vi "Write Wavelength.vi"(8 "error in":errorcluster, 10 "Wavelength (nm)":dbl, 11 "LTB-1 in":refnum<class "LTB-1.lvclass">) -> (0 "error out":errorcluster, 3 "LTB-1 out":refnum<class "LTB-1.lvclass">)   [LabVIEW 2018, in "LTB-1.lvlib" / "LTB-1.lvclass"]
doc: "This is an override VI, call parent method before or after child method overrites it. Write the target wavelength to the EXFO. For Luminar the wavelength should be 1550 nm. If there is a tolerance, make sure it does not exceed +-5 nm or we risk violating ITAR\n\nAuthor: Ron Dexter\nCompany: Luminar\nModified: 5/20/2018"
uses:
  LTB-1.lvclass
  C:/AME Test Engineering/LabVIEW/PPLs/EXFO/Parent/EXFO.lvlibp/EXFO.lvclass
  LTB-1.lvclass/LTB-1.ctl
  PPLs/EXFO/Parent/EXFO.lvlibp/Methods/Read Resource.vi
  3150 Driver/3150.lvlib
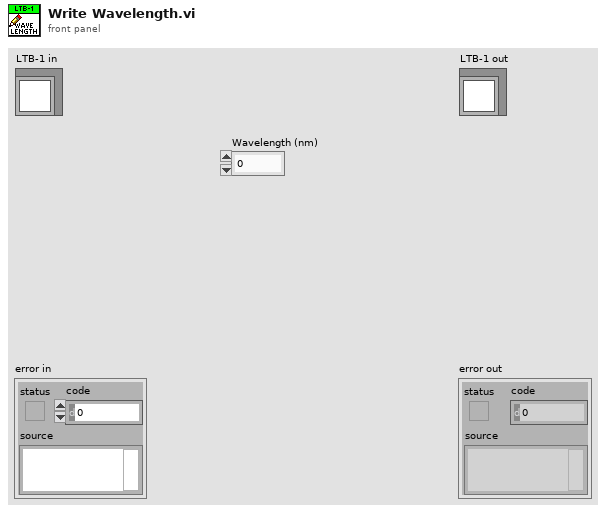
[diagram p1: front panel]
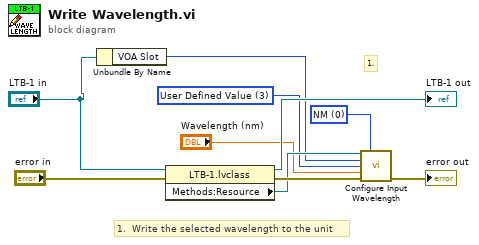
[diagram p0: block diagram]
diagram:
  w5 = u16 0 items=["NM", "M"] ("Wavelength Unit (0:NM)")
  w2 = 3 items=["MINimum", "MAXimum", "DEFault", "User Defined Value"] ("Wavelength (0:MINimum)")
  # "1.  Write the selected wavelength to the unit"
  # "1."
  n1 = Unbundle By Name("LTB-1 in") -> ("VOA Slot"=w3:i16)
  n2 = property class="LTB-1.lvclass"(reference="LTB-1 in", error in="error in") -> (reference out=→"LTB-1 out":refnum<class "LTB-1.lvclass">, error out=w6:errorcluster, "Methods:Resource"=w4:refnum<visa-resource-name>)
  n3 = call "Configure Input Wavelength.vi"("VISA resource name"=w4, "Wavelength Unit (0:NM)"=w5, "Platform Slot Number (10)"=w3, "Wavelength (0:MINimum)"=w2, "User Defined Wavelength Value (1310)"="Wavelength (nm)", "error in (no error)"=w6) -> ("error out"=→"error out":errorcluster)  [unwired: 8 in, 1 out]
